vi "MaxI64.vi"() -> (0 "Maximum value":i64)   [LabVIEW 2017, in "GPNumeric.lvlib"]
doc: "Returns the <B>Maximum value</B> of the given data type.\n\nThis VI is inlined and thus just as fast as an ordinary constant dropped on the block diagram, but it documents this specific value better than even a labeled constant does.\n\nSteen Schmidt\nGPower\n16/5 2014"
uses:
  GPNumeric.lvlib
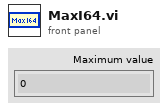
[diagram p1: front panel]
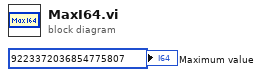
[diagram p0: block diagram]
diagram:
  "Maximum value" <- i64 9223372036854775807
